vi "Ramp Vector String, New.vi"(1 "step (1)":i32=1, 2 "nelem":i32=5, 3 "start (0)":i32) -> (0 "ramp":string[](array[string]))   [LabVIEW 2010]
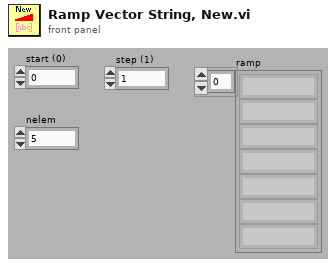
[diagram p1: front panel]
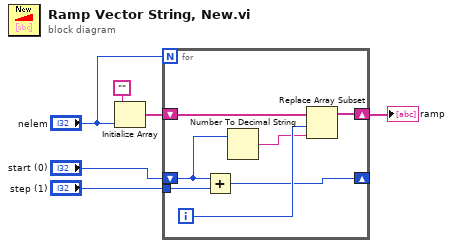
[diagram p0: block diagram]
diagram:
  n1 = Initialize Array("", "nelem") -> (w6:string[])
  n2 = for {
    N: "nelem" -> [_]
    shift-right: [w13] -> w5
    shift-left: w6 -> [w12]
    shift-right: [w7] -> _
    shift-left: "start (0)" -> [w8]
    tunnel: "step (1)" -> [w10]
    i -> [w11]
    n3 = Add(x=w8, y=w10) -> (x+y=w7:i32)
    n4 = Number To Decimal String(number=w8) -> (decimal integer string=w9:string)  [unwired: 1 in]
    n5 = Replace Array Subset(array=w12, new element=w9, index=w11) -> (w13:string[])
  }
  "ramp" <- w5
